vi "BuildTerrain.vi"() -> ()   [LabVIEW 2010]
uses:
  <vilib>/Utility/miscctls.llb/LVPoint32TypeDef.ctl
  <vilib>/Utility/miscctls.llb/LV3DPointTypeDef.ctl
  <vilib>/picture/3D Picture Control/NI_3D Picture Control.lvlib
panel:
  in  "vert":dbl(slide) scale=0.0..2.0
  in  "Horiz":dbl(slide) scale=0.0..2.0
  out "Coords":T1
  out "stage":refnum<vi>(3d-picture)
  in  "done":bool
  in  "Zoom":dbl(slide) scale=0.1..1.0
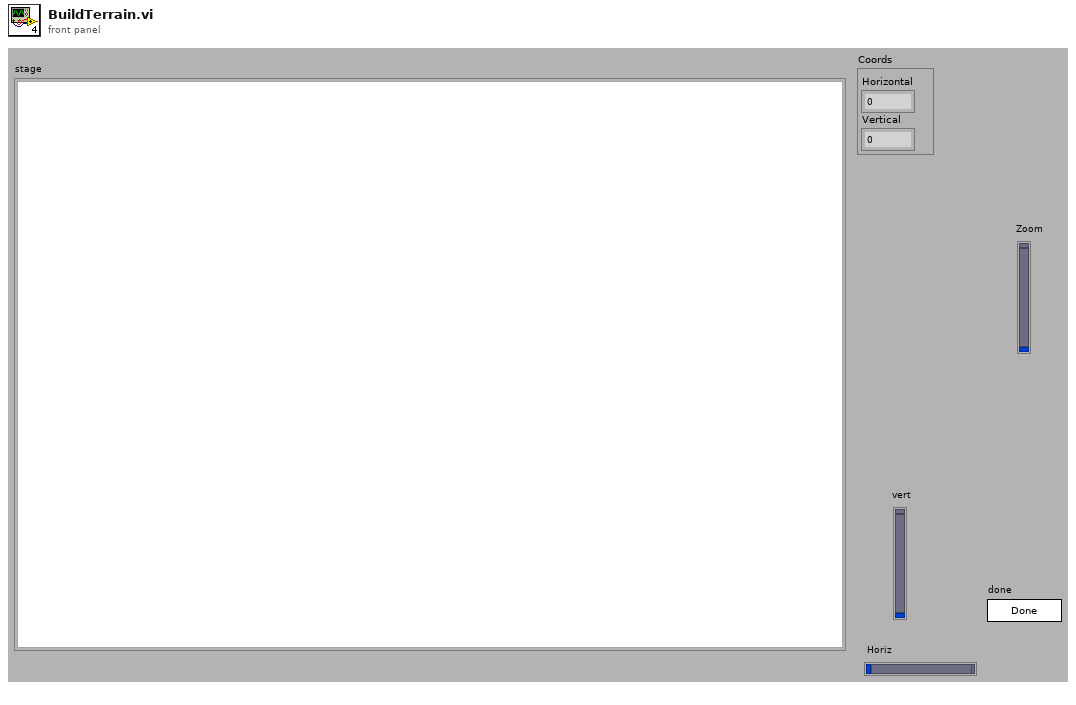
[diagram p1: front panel]
types:
  T1 = typedef "LVPoint32TypeDef.ctl" = cluster{"Horizontal":i32, "Vertical":i32}
  T2 = typedef "LV3DPointTypeDef.ctl" = cluster{"X":sgl, "Y":sgl, "Z":sgl}
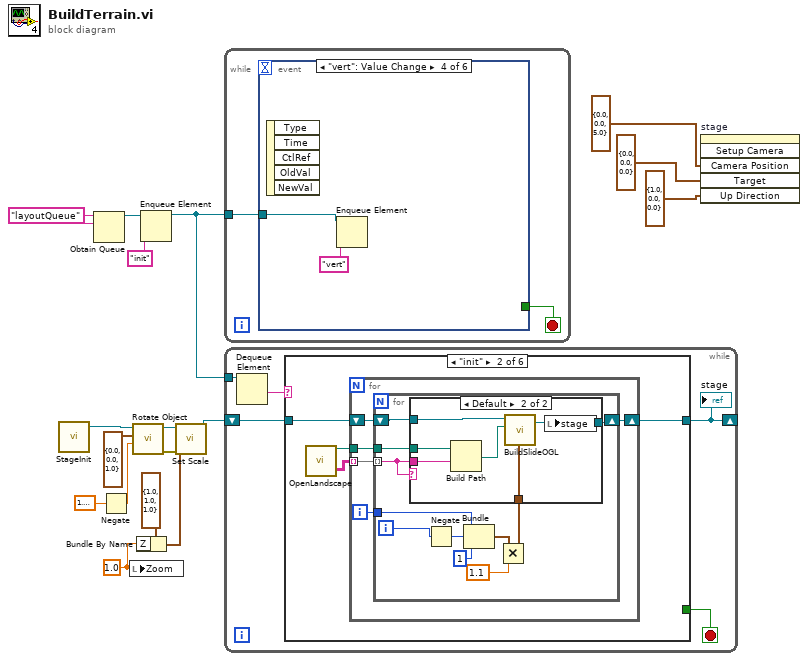
[diagram p0: block diagram]
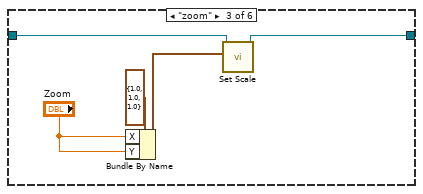
[diagram p4: hidden frame]
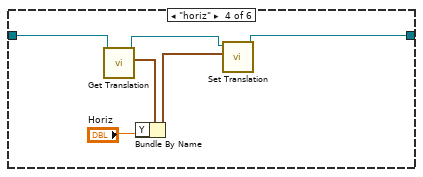
[diagram p5: hidden frame]
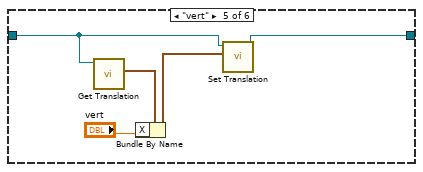
[diagram p6: hidden frame]
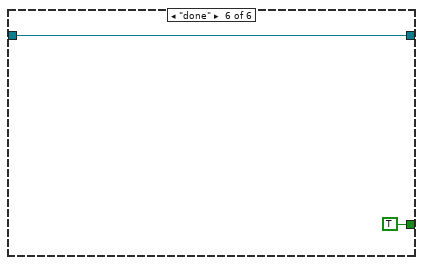
[diagram p7: hidden frame]
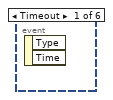
[diagram p8: hidden frame]
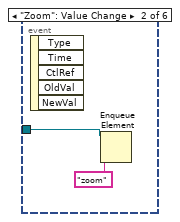
[diagram p9: hidden frame]
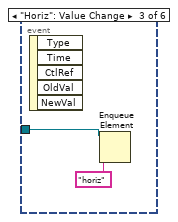
[diagram p10: hidden frame]
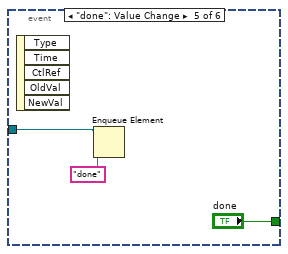
[diagram p11: hidden frame]
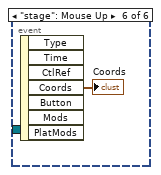
[diagram p12: hidden frame]
diagram:
  w3 = sgl 1.0 ("Zoom Factor")
  w16 = "layoutQueue" ("name (unnamed)")
  n1 = call <userlib>:"StageInit.vi"() -> ("Stage out"=w10:refnum<vi>)  [unwired: 4 in, 1 out]
  n2 = Obtain Queue(name (unnamed)=w16, element data type=w16) -> (queue out=w17:refnum<queue>)  [unwired: 3 in, 2 out]
  n3 = Negate(x=1.5707963267948966) -> (-x=w9:dbl)
  n4 = local write "Zoom"(w3) -> ()
  n5 = call <vilib>:"Rotate Object.vi"("Angle"=w9, "Axis"=cluster{"X":sgl, "Y":sgl, "Z":sgl} {"X"=0.0, "Y"=0.0, "Z"=1.0}, "Scene.Object In"=w10) -> ("error out"=w6:errorcluster, "Scene.Object Out"=w5:refnum<vi>)  [unwired: 7 in]
  n6 = Bundle By Name(cluster=cluster{"X":sgl, "Y":sgl, "Z":sgl} {"X"=1.0, "Y"=1.0, "Z"=1.0} ("Axis"), "Z"=w3) -> (w1:cluster{"X":sgl, "Y":sgl, "Z":sgl})
  n7 = Enqueue Element(queue=w17, element="init") -> (queue out=w14:refnum<queue>)  [unwired: 2 in, 2 out]
  n8 = call <vilib>:"Set Scale.vi"("error in (no error)"=w6, "Scale"=w1, "Scene Object"=w5) -> ("Scaled Object"=w4:refnum<vi>)  [unwired: 7 in, 1 out]
  n9 = while {
    tunnel: w14 -> [w18]
    stop <- w19 stop-if-true
    n10 = event shown="[3] \"vert\": Value Change" {
      selector: _ -> [_ _ _ _ _ _]
      dyn-events: _ -> [_ _ _ _ _ _]
      timeout: _ -> [_ _ _ _ _ _]
      tunnel: [_ _ _ _ "done" _] -> w19
      tunnel: w18 -> [_ w20 w22 w24 w26 _]
      event Timeout {
        n11 = event-data() -> ()  [unwired: 1 in, 2 out]
      }
      event "Zoom": Value Change {
        n12 = event-data() -> ()  [unwired: 1 in, 5 out]
        n13 = Enqueue Element(queue=w20, element="zoom") -> ()  [unwired: 2 in, 3 out]
      }
      event "Horiz": Value Change {
        n14 = event-data() -> ()  [unwired: 1 in, 5 out]
        n15 = Enqueue Element(queue=w22, element="horiz") -> ()  [unwired: 2 in, 3 out]
      }
      event "vert": Value Change {
        n16 = event-data() -> ()  [unwired: 1 in, 5 out]
        n17 = Enqueue Element(queue=w24, element="vert") -> ()  [unwired: 2 in, 3 out]
      }
      event "done": Value Change {
        n18 = event-data() -> ()  [unwired: 1 in, 5 out]
        n19 = Enqueue Element(queue=w26, element="done") -> ()  [unwired: 2 in, 3 out]
      }
      event "stage": Mouse Up {
        n20 = event-data() -> ("Coords"=→"Coords":T1)  [unwired: 1 in, 6 out]
      }
    }
  }
  n21 = while {
    tunnel: w14 -> [w34]
    shift-right: [w30] -> _
    shift-left: w4 -> [w31]
    stop <- w32 stop-if-true
    n22 = Dequeue Element(queue=w34) -> (element=w33:string)  [unwired: 2 in, 3 out]
    n23 = case shown="\"init\"" w33 {
      tunnel: [_ _ _ _ _ TRUE] -> w32
      tunnel: w31 -> [w35 w39 w66 w70 w75 w79]
      tunnel: [w35 w38 w64 w72 w78 w79] -> w30
      frame Default {
      }
      frame "init" {
        n24 = call "OpenLandscape.vi"() -> ("Landscape"=w37:string[][], "Slides"=w36:path)  [unwired: 1 in]
        n25 = for {
          shift-right: [w43] -> w38
          shift-left: w39 -> [w44]
          tunnel: w37 -> [w42] mode=indexing
          tunnel: w36 -> [w41]
          i -> [w40]
          n26 = for {
            shift-right: [w51] -> w43
            shift-left: w44 -> [w55]
            tunnel: w42 -> [w45] mode=indexing
            tunnel: w41 -> [w50]
            tunnel: w40 -> [w49]
            i -> [w48]
            n27 = Negate(x=w48) -> (-x=w52:i32)
            n28 = Bundle(w49, w52, "y"=1) -> (w47:cluster{i32, i32, "y":i32})  [unwired: 1 in]
            n29 = Multiply(x=w47, y=1.1) -> (x*y=w46:cluster{dbl, dbl, "y":dbl})
            n30 = case shown="Default" w45 {
              tunnel: w55 -> [w56 w62]
              tunnel: [w56 w60] -> w51
              tunnel: w45 -> [_ w59]
              tunnel: w50 -> [_ w58]
              tunnel: w46 -> [_ w57]
              frame "" {
              }
              frame Default {
                n31 = Build Path(base path=w58, name or relative path=w59) -> (appended path=w61:path)
                n32 = call "BuildSlideOGL.vi"("Translation"=w57, "slide"=w61, "Stage In"=w62) -> ("Stage out"=w60:refnum<vi>)  [unwired: 1 in, 1 out]
                n33 = local write "stage"(w60) -> ()
              }
            }
          }
        }
      }
      frame "zoom" {
        n34 = Bundle By Name(cluster=cluster{"X":sgl, "Y":sgl, "Z":sgl} {"X"=1.0, "Y"=1.0, "Z"=1.0} ("Axis"), "X"="Zoom", "Y"="Zoom") -> (w65:cluster{"X":sgl, "Y":sgl, "Z":sgl})
        n35 = call <vilib>:"Set Scale.vi"("Scale"=w65, "Scene Object"=w66) -> ("Scaled Object"=w64:refnum<vi>)  [unwired: 8 in, 1 out]
      }
      frame "horiz" {
        n36 = call <vilib>:"Get Translation.vi"("Scene Object"=w70) -> ("Transformation:Get Translation"=w71:cluster{"X":sgl, "Y":sgl, "Z":sgl}, "Scene Object"=w69:refnum<vi>)  [unwired: 8 in, 1 out]
        n37 = Bundle By Name(cluster=w71, "Y"="Horiz") -> (w73:cluster{"X":sgl, "Y":sgl, "Z":sgl})
        n38 = call <vilib>:"Set Translation.vi"("Translation"=w73, "Scene Object"=w69) -> ("Translated Object"=w72:refnum<vi>)  [unwired: 8 in, 1 out]
      }
      frame "vert" {
        n39 = call <vilib>:"Get Translation.vi"("Scene Object"=w75) -> ("Transformation:Get Translation"=w74:cluster{"X":sgl, "Y":sgl, "Z":sgl})  [unwired: 8 in, 2 out]
        n40 = Bundle By Name(cluster=w74, "X"="vert") -> (w77:cluster{"X":sgl, "Y":sgl, "Z":sgl})
        n41 = call <vilib>:"Set Translation.vi"("Translation"=w77, "Scene Object"=w75) -> ("Translated Object"=w78:refnum<vi>)  [unwired: 8 in, 1 out]
      }
      frame "done" {
      }
    }
    "stage" <- w30
  }
  n42 = invoke on="stage" class="SceneGraphDisp (strict)" method="Setup Camera"("Camera Position"=T2 {"X"=0.0, "Y"=0.0, "Z"=5.0}, "Target"=T2 {"X"=0.0, "Y"=0.0, "Z"=0.0}, "Up Direction"=T2 {"X"=1.0, "Y"=0.0, "Z"=0.0}) -> ()  [unwired: 3 in, 6 out]
